vi "Temp Control.vi"() -> ()   [LabVIEW 2015]
uses:
  <vilib>/addons/control/pid/NI_PID_autopid.lvlib
  <vilib>/addons/control/pid/autopid.llb/PID Online Autotuning (Relay Feedback).vi
  <vilib>/addons/control/pid/NI_PID_pid.lvlib
  <vilib>/addons/control/pid/pid.llb/PID Control Input Filter (DBL).vi
  <vilib>/MakerHub/LINX/LMH-LINX.lvlib
  <vilib>/ni845x/ni845x.llb/ni845xControl.ctl
panel:
  in  "IR Sensor Device":T1
  in  "Arduino COMM Port":refnum<visa-resource-name>
  out "error out":errorcluster
  out "Temperature 7":dbl format="%#_g'C"
  out "Temperature 2":dbl format="%#_g'C"
  out "Temperature 6":dbl format="%#_g'C"
  out "Temperature 3":dbl format="%#_g'C"
  out "Temperature 1":dbl format="%#_g'C"
  out "Teperature Chart":T2(graph)
  out "Temp SS? 5":bool=TRUE
  in  "Temperature Control 5":bool=TRUE
  in  "Temperature  5":dbl format="%#_g'C"
  out "Temperature 5":dbl format="%#_g'C"
  in  "SSR Duration 5":dbl
  out "Temp SS? 4":bool=TRUE
  in  "Temperature Control 4":bool=TRUE
  in  "Temperature  4":dbl format="%#_g'C"
  out "Temperature 4":dbl format="%#_g'C"
  in  "SSR Duration 4":dbl
  out "Flowrate Sensor 2":dbl format="%#_13g"
  out "Flowrate Sensor 1":dbl format="%#_13g"
  out "Pressure 2":dbl format="%#_13g"
  out "Pressure 1":dbl format="%#_13g"
  in  "Stop":bool=TRUE
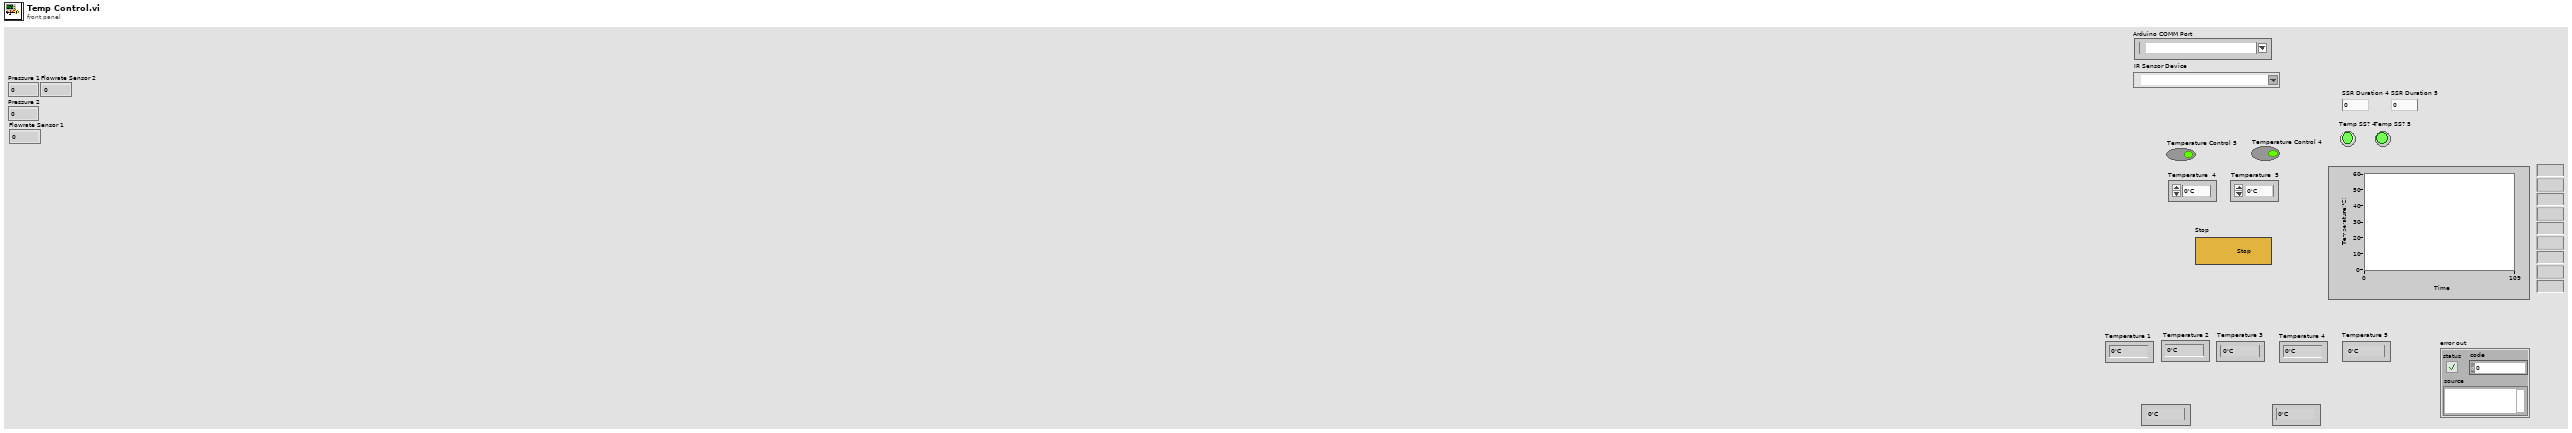
[diagram p1: front panel]
types:
  T1 = typedef "ni845xControl.ctl" = refnum<k21>
  T2 = cluster{"[0]":dbl, "[1]":dbl, "[2]":dbl, "[3]":dbl, "[4]":dbl, "[5]":dbl, "[6]":dbl, "[7]":dbl, "[8]":dbl}
  T3 = typedef "LMH-LINX.lvlib/LINX Ref.ctl" = cluster{"Platform":T4, "Interface":T5, "LINX Device Config":T6}
  T4 = typedef "LMH-LINX.lvlib/Platform.ctl" = enum16{"LINX", "myRIO"}
  T5 = typedef "LMH-LINX.lvlib/Interface.ctl" = enum16{"Serial", "TCP"}
  T6 = typedef "LMH-LINX.lvlib/Device.lvlib/LINX Device Config.ctl" = cluster{"Interface":T5, "COM Port":refnum<visa-resource-name>, "TCP Configuration":T7, "Device Family":u8, "Device ID":u8, "Device Name":string, "TCP Ref":refnum<k5>, "Channels":T8}
  T7 = typedef "LMH-LINX.lvlib/Device.lvlib/TCP Config.ctl" = cluster{"IP Address":string, "Port":u16}
  T8 = typedef "LMH-LINX.lvlib/Channels.ctl" = cluster{"DI":u8[], "DO":u8[], "AI":u8[], "AO":u8[], "PWM":u8[], "QE":u8[], "UART":u8[], "I2C 2":u8[], "SPI":u8[], "CAN":u8[], "Servo":u8[], "AI Ref (V)":dbl, "AO Ref (V)":dbl, "AO Resolution (Bits)":u8}
  T9 = cluster{"Proportional gain Kc":dbl, "Integral time Ti (sec)":dbl, "Derivative time Ti (sec)":dbl}
  T10 = cluster{"type of controller":enum16{"P", "PI", "PID"}, "relay cycles":i32, "relay amplitude":dbl, "control specifications":enum16{"Fast", "Normal", "Slow"}, "PV noise level":dbl}
  T11 = cluster{"proportional gain (Kc)":dbl, "integral time (Ti, min)":dbl, "derivative time (Td, min)":dbl}
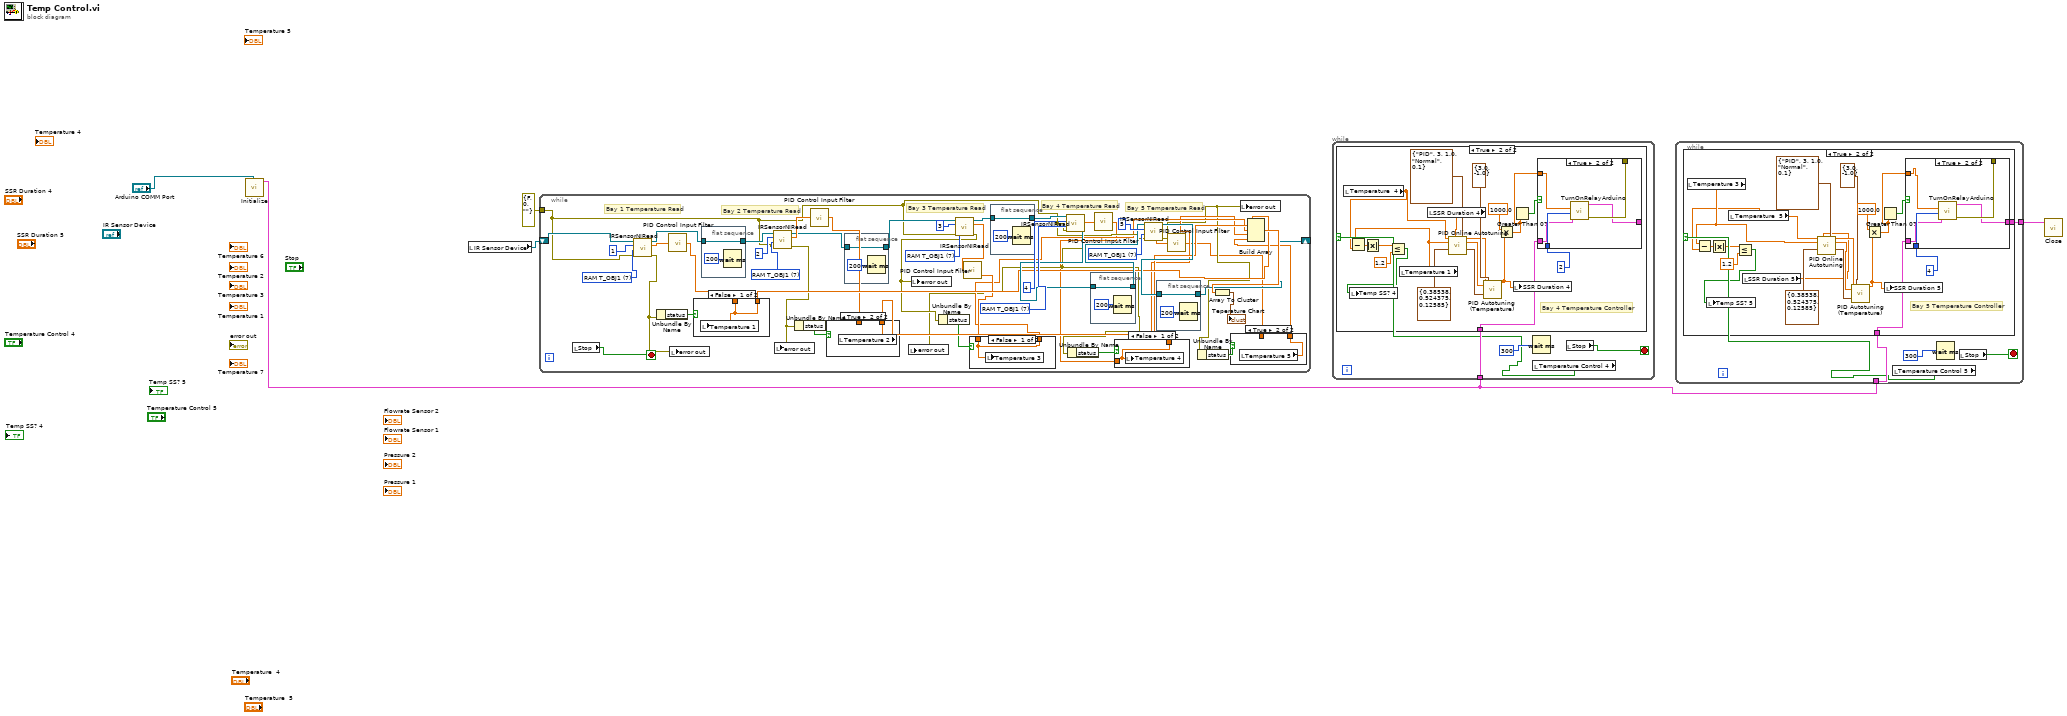
[diagram p0: block diagram]
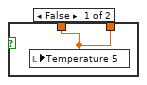
[diagram p2: hidden frame]
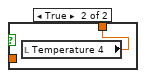
[diagram p3: hidden frame]
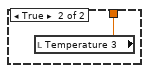
[diagram p4: hidden frame]
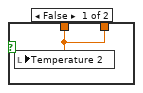
[diagram p5: hidden frame]
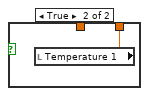
[diagram p6: hidden frame]
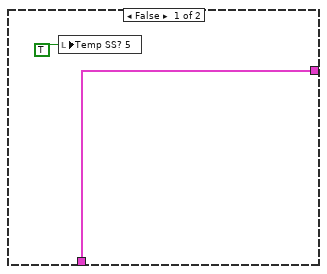
[diagram p7: hidden frame]
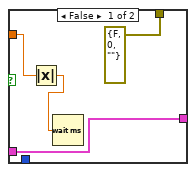
[diagram p8: hidden frame]
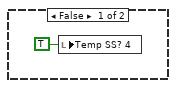
[diagram p9: hidden frame]
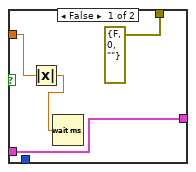
[diagram p10: hidden frame]
diagram:
  n1 = call <vilib>:"Initialize.vi"("Serial Port"="Arduino COMM Port") -> ("LINX Ref"=w3:T3)  [unwired: 8 in, 2 out]
  n2 = local read "IR Sensor Device"() -> (w2:T1)
  n3 = while {
    shift-right: [w27] -> _
    shift-left: w2 -> [w28]
    tunnel: errorcluster {"status"=FALSE, "code"=0, "source"=""} ("error out") -> [w26]
    stop <- w52 stop-if-true
    w43 = u8 7 items=["RAM IR raw  Ch1"=4, "RAM IR raw  Ch2"=5, "RAM T_A"=6, "RAM T_OBJ1"=7, "RAM T_OBJ2"=8, "EEPROM_To_max"=32, "EEPROM_To_min"=33, "EEPROM_PWM_CTRL"=34, "EEPROM_Ta_range"=35, "EEPROM_Emissivity_CorrCoeff"=36, "EEPROM_SMBus Address"=46, "EEPROM_ConfigReg"=37] ("Melexis_Cmmds")
    w45 = u8 7 items=["RAM IR raw  Ch1"=4, "RAM IR raw  Ch2"=5, "RAM T_A"=6, "RAM T_OBJ1"=7, "RAM T_OBJ2"=8, "EEPROM_To_max"=32, "EEPROM_To_min"=33, "EEPROM_PWM_CTRL"=34, "EEPROM_Ta_range"=35, "EEPROM_Emissivity_CorrCoeff"=36, "EEPROM_SMBus Address"=46, "EEPROM_ConfigReg"=37] ("Melexis_Cmmds")
    w44 = u8 7 items=["RAM IR raw  Ch1"=4, "RAM IR raw  Ch2"=5, "RAM T_A"=6, "RAM T_OBJ1"=7, "RAM T_OBJ2"=8, "EEPROM_To_max"=32, "EEPROM_To_min"=33, "EEPROM_PWM_CTRL"=34, "EEPROM_Ta_range"=35, "EEPROM_Emissivity_CorrCoeff"=36, "EEPROM_SMBus Address"=46, "EEPROM_ConfigReg"=37] ("Melexis_Cmmds")
    w49 = u8 7 items=["RAM IR raw  Ch1"=4, "RAM IR raw  Ch2"=5, "RAM T_A"=6, "RAM T_OBJ1"=7, "RAM T_OBJ2"=8, "EEPROM_To_max"=32, "EEPROM_To_min"=33, "EEPROM_PWM_CTRL"=34, "EEPROM_Ta_range"=35, "EEPROM_Emissivity_CorrCoeff"=36, "EEPROM_SMBus Address"=46, "EEPROM_ConfigReg"=37] ("Melexis_Cmmds")
    w54 = u8 7 items=["RAM IR raw  Ch1"=4, "RAM IR raw  Ch2"=5, "RAM T_A"=6, "RAM T_OBJ1"=7, "RAM T_OBJ2"=8, "EEPROM_To_max"=32, "EEPROM_To_min"=33, "EEPROM_PWM_CTRL"=34, "EEPROM_Ta_range"=35, "EEPROM_Emissivity_CorrCoeff"=36, "EEPROM_SMBus Address"=46, "EEPROM_ConfigReg"=37] ("Melexis_Cmmds")
    # "Bay 5 Temperature Read"
    # "Bay 4 Temperature Read"
    # "Bay 3 Temperature Read"
    # "Bay 2 Temperature Read"
    # "Bay 1 Temperature Read"
    n4 = local read "Stop"() -> (w52:bool)
    n5 = call "IRSensorNIRead.vi"("error in (no error)"=w26, "Melexis_Cmmds"=w54, "Address"=u8 1, "device reference"=w28) -> ("error out"=w25:errorcluster, "Temperature"=w55:dbl, "device reference out"=w51:T1)  [unwired: 5 in]
    n6 = Unbundle By Name(w25) -> ("status"=w24:bool)
    n7 = call-poly <vilib>:"PID Control Input Filter.vi"("input"=w55) -> ("output"=w23:dbl)  [unwired: 4 in]
    n8 = local write "error out"(w25) -> ()
    n9 = case shown="False" w24 {
      tunnel: w23 -> [w64 _]
      tunnel: [w64 w65] -> w22
      frame False {
        n10 = local write "Temperature 1"(w64) -> ()
      }
      frame True {
        n11 = local read "Temperature 1"() -> (w65:dbl)
      }
    }
    n12 = flat-sequence {
      tunnel: w51 -> [w74]
      tunnel: [w74] -> w50
      frame #0 {
        n13 = Wait (ms)(milliseconds to wait=u32 200) -> ()  [unwired: 1 out]
      }
    }
    n14 = call "IRSensorNIRead.vi"("error in (no error)"=w26, "Melexis_Cmmds"=w49, "Address"=u8 2, "device reference"=w50) -> ("error out"=w21:errorcluster, "Temperature"=w47:dbl, "device reference out"=w46:T1)  [unwired: 5 in]
    n15 = local write "error out"(w21) -> ()
    n16 = Unbundle By Name(w21) -> ("status"=w20:bool)
    n17 = call-poly <vilib>:"PID Control Input Filter.vi"("input"=w47) -> ("output"=w19:dbl)  [unwired: 4 in]
    n18 = case shown="True" w20 {
      tunnel: w19 -> [w62 _]
      tunnel: [w62 w63] -> w18
      frame False {
        n19 = local write "Temperature 2"(w62) -> ()
      }
      frame True {
        n20 = local read "Temperature 2"() -> (w63:dbl)
      }
    }
    n21 = flat-sequence {
      tunnel: w46 -> [w72]
      tunnel: [w72] -> w39
      frame #0 {
        n22 = Wait (ms)(milliseconds to wait=u32 200) -> ()  [unwired: 1 out]
      }
    }
    n23 = call "IRSensorNIRead.vi"("error in (no error)"=w26, "Melexis_Cmmds"=w44, "Address"=u8 3, "device reference"=w39) -> ("error out"=w14:errorcluster, "Temperature"=w34:dbl, "device reference out"=w38:T1)  [unwired: 5 in]
    n24 = local write "error out"(w14) -> ()
    n25 = Unbundle By Name(w14) -> ("status"=w15:bool)
    n26 = call-poly <vilib>:"PID Control Input Filter.vi"("input"=w34) -> ("output"=w17:dbl)  [unwired: 4 in]
    n27 = case shown="False" w15 {
      tunnel: w17 -> [w60 _]
      tunnel: [w60 w61] -> w16
      frame False {
        n28 = local write "Temperature 3"(w60) -> ()
      }
      frame True {
        n29 = local read "Temperature 3"() -> (w61:dbl)
      }
    }
    n30 = flat-sequence {
      tunnel: w38 -> [w70]
      tunnel: [w70] -> w36
      frame #0 {
        n31 = Wait (ms)(milliseconds to wait=u32 200) -> ()  [unwired: 1 out]
      }
    }
    n32 = call "IRSensorNIRead.vi"("error in (no error)"=w26, "Melexis_Cmmds"=w45, "Address"=u8 4, "device reference"=w36) -> ("error out"=w13:errorcluster, "Temperature"=w33:dbl, "device reference out"=w37:T1)  [unwired: 5 in]
    n33 = local write "error out"(w13) -> ()
    n34 = Unbundle By Name(w13) -> ("status"=w11:bool)
    n35 = flat-sequence {
      tunnel: w37 -> [w68]
      tunnel: [w68] -> w35
      frame #0 {
        n36 = Wait (ms)(milliseconds to wait=u32 200) -> ()  [unwired: 1 out]
      }
    }
    n37 = call-poly <vilib>:"PID Control Input Filter.vi"("input"=w33) -> ("output"=w12:dbl)  [unwired: 4 in]
    n38 = case shown="False" w11 {
      tunnel: w12 -> [w58 _]
      tunnel: [w58 w59] -> w10
      frame False {
        n39 = local write "Temperature 4"(w58) -> ()
      }
      frame True {
        n40 = local read "Temperature 4"() -> (w59:dbl)
      }
    }
    n41 = call "IRSensorNIRead.vi"("error in (no error)"=w26, "Melexis_Cmmds"=w43, "Address"=u8 5, "device reference"=w35) -> ("error out"=w9:errorcluster, "Temperature"=w32:dbl, "device reference out"=w31:T1)  [unwired: 5 in]
    n42 = flat-sequence {
      tunnel: w31 -> [w66]
      tunnel: [w66] -> w27
      frame #0 {
        n43 = Wait (ms)(milliseconds to wait=u32 200) -> ()  [unwired: 1 out]
      }
    }
    n44 = call-poly <vilib>:"PID Control Input Filter.vi"("input"=w32) -> ("output"=w7:dbl)  [unwired: 4 in]
    n45 = Unbundle By Name(w9) -> ("status"=w8:bool)
    n46 = case shown="True" w8 {
      tunnel: w7 -> [w56 _]
      tunnel: [w56 w57] -> w6
      frame False {
        n47 = local write "Temperature 5"(w56) -> ()
      }
      frame True {
        n48 = local read "Temperature 5"() -> (w57:dbl)
      }
    }
    n49 = local write "error out"(w9) -> ()
    n50 = Build Array(w22, w18, w16, w10, w6) -> (w30:dbl[])
    n51 = Array To Cluster(array=w30) -> (cluster=→"Teperature Chart":T2)
  }
  n52 = while {
    tunnel: w3 -> [w78]
    stop <- w77 stop-if-true
    n53 = Wait (ms)(milliseconds to wait=u32 300) -> ()  [unwired: 1 out]
    n54 = local read "Temperature Control 4"() -> (w76:bool)
    n55 = case shown="True" w76 {
      tunnel: w78 -> [_ w98]
      frame False {
        n56 = local write "Temp SS? 4"(TRUE ("Temp SS? 4")) -> ()
      }
      frame True {
        # "Bay 4 Temperature Controller"
        n57 = local read "Temperature  4"() -> (w81:dbl)
        n58 = local read "Temperature 1"() -> (w82:dbl)
        n59 = Subtract(x=w82, y=w81) -> (x-y=w84:dbl)
        n60 = Absolute Value(x=w84) -> (abs(x)=w86:dbl)
        n61 = Less Or Equal?(x=w86, y=1.2) -> (x <= y?=w83:bool)
        n62 = local write "Temp SS? 4"(w83) -> ()
        n63 = local read "SSR Duration 4"() -> (w87:dbl)
        n64 = call-poly <vilib>:"PID Online Autotuning.vi"("setpoint"=w81, "manipulated variable"=w87, "autotuning parameters"=T10 {"type of controller"=enum."PID", "relay cycles"=3, "relay amplitude"=1.0, "control specifications"=enum."Normal", "PV noise level"=0.1} ("Autotuning Parameters R1"), "process variable"=w82, "PID gains in"=T9 {"Proportional gain Kc"=0.38538, "Integral time Ti (sec)"=0.524375, "Derivative time Ti (sec)"=0.12585} ("PID gains 2")) -> ("setpoint out"=w89:dbl, "process variable out"=w90:dbl, "PID gains out"=w92:T11)  [unwired: 6 in, 2 out]
        n65 = call <vilib>:"PID Autotuning (Temperature).vi"("desired temperature"=w89, "measured temperature"=w90, "PID gains in"=w92, "output range"=cluster{"output high":dbl, "output low":dbl} {"output high"=3.0, "output low"=-1.0} ("Output range")) -> ("output"=w88:dbl)  [unwired: 12 in, 3 out]
        n66 = Multiply(x=1000.0, y=w88) -> (x*y=w96:dbl)
        n67 = Greater Than 0?(x=w96) -> (x > 0?=w97:bool)
        n68 = local write "SSR Duration 4"(w88) -> ()
        n69 = case shown="True" w97 {
          tunnel: [errorcluster {"status"=FALSE, "code"=0, "source"=""} ("error out") w107] -> _
          tunnel: 2 -> [_ w108]
          tunnel: [w101 w106] -> _
          tunnel: w98 -> [w101 w105]
          tunnel: w96 -> [w100 w104]
          frame False {
            n70 = Absolute Value(x=w100) -> (abs(x)=w102:dbl)
            n71 = Wait (ms)(milliseconds to wait=w102) -> ()  [unwired: 1 out]
          }
          frame True {
            n72 = call "TurnOnRelayArduino.vi"("channel"=w108, "duration"=w104, "LINX Resource"=w105) -> ("error out"=w107:errorcluster, "LINX Resource Out"=w106:T3)  [unwired: 7 in]
          }
        }
      }
    }
    n73 = local read "Stop"() -> (w77:bool)
  }
  n74 = while {
    tunnel: w3 -> [w111]
    tunnel: [w109] -> w1
    stop <- w112 stop-if-true
    n75 = local read "Temperature Control 5"() -> (w110:bool)
    n76 = case shown="True" w110 {
      tunnel: w111 -> [w114 w134]
      tunnel: [w114 w116] -> w109
      frame False {
        n77 = local write "Temp SS? 5"(TRUE ("Temp SS? 5")) -> ()
      }
      frame True {
        # "Bay 5 Temperature Controller"
        n78 = local read "Temperature 3"() -> (w118:dbl)
        n79 = local read "Temperature  5"() -> (w117:dbl)
        n80 = Subtract(x=w118, y=w117) -> (x-y=w120:dbl)
        n81 = Absolute Value(x=w120) -> (abs(x)=w122:dbl)
        n82 = Less Or Equal?(x=w122, y=1.2) -> (x <= y?=w119:bool)
        n83 = local write "Temp SS? 5"(w119) -> ()
        n84 = local read "SSR Duration 5"() -> (w123:dbl)
        n85 = call-poly <vilib>:"PID Online Autotuning.vi"("setpoint"=w117, "manipulated variable"=w123, "autotuning parameters"=T10 {"type of controller"=enum."PID", "relay cycles"=3, "relay amplitude"=1.0, "control specifications"=enum."Normal", "PV noise level"=0.1} ("Autotuning Parameters R1"), "process variable"=w118, "PID gains in"=T9 {"Proportional gain Kc"=0.38538, "Integral time Ti (sec)"=0.524375, "Derivative time Ti (sec)"=0.12585} ("PID gains 2")) -> ("setpoint out"=w125:dbl, "process variable out"=w126:dbl, "PID gains out"=w128:T11)  [unwired: 6 in, 2 out]
        n86 = call <vilib>:"PID Autotuning (Temperature).vi"("desired temperature"=w125, "measured temperature"=w126, "PID gains in"=w128, "output range"=cluster{"output high":dbl, "output low":dbl} {"output high"=3.0, "output low"=-1.0} ("Output range")) -> ("output"=w124:dbl)  [unwired: 12 in, 3 out]
        n87 = Multiply(x=1000.0, y=w124) -> (x*y=w132:dbl)
        n88 = Greater Than 0?(x=w132) -> (x > 0?=w133:bool)
        n89 = local write "SSR Duration 5"(w124) -> ()
        n90 = case shown="True" w133 {
          tunnel: [errorcluster {"status"=FALSE, "code"=0, "source"=""} ("error out") w143] -> _
          tunnel: 4 -> [_ w144]
          tunnel: [w137 w142] -> w116
          tunnel: w134 -> [w137 w141]
          tunnel: w132 -> [w136 w140]
          frame False {
            n91 = Absolute Value(x=w136) -> (abs(x)=w138:dbl)
            n92 = Wait (ms)(milliseconds to wait=w138) -> ()  [unwired: 1 out]
          }
          frame True {
            n93 = call "TurnOnRelayArduino.vi"("channel"=w144, "duration"=w140, "LINX Resource"=w141) -> ("error out"=w143:errorcluster, "LINX Resource Out"=w142:T3)  [unwired: 7 in]
          }
        }
      }
    }
    n94 = Wait (ms)(milliseconds to wait=u32 300) -> ()  [unwired: 1 out]
    n95 = local read "Stop"() -> (w112:bool)
  }
  n96 = call <vilib>:"Close.vi"("LINX Resource"=w1) -> ()  [unwired: 9 in, 2 out]
